vi "WebDAV write.vi"(0 "RIO Filepath":path, 5 "CA Number":string, 7 "Test Name":string, 9 "Date":string, 11 "Filename":string) -> (15 "error out":errorcluster)   [LabVIEW 2019]
uses:
  <vilib>/WebDAVClient/Advanced/Put File.vi
  <vilib>/WebDAVClient/NI_WebDAV.lvlib
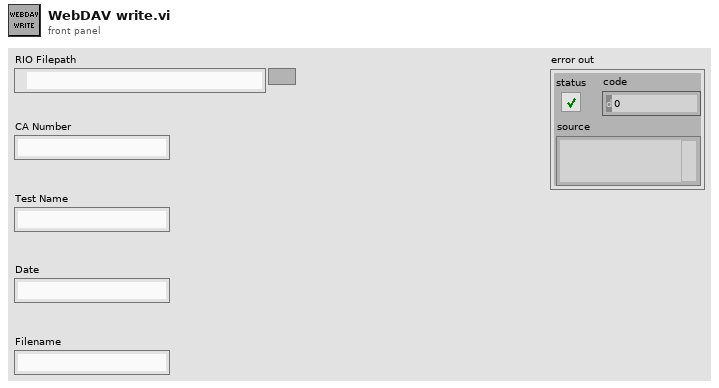
[diagram p1: front panel]
types:
  T1 = typedef "NI_WebDAV.lvlib/SessionHandle.ctl" = refnum<k1>
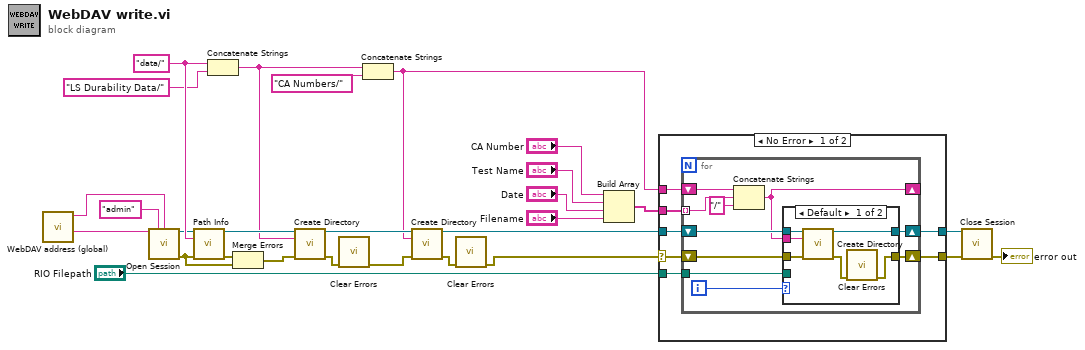
[diagram p0: block diagram]
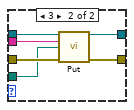
[diagram p2: hidden frame]
diagram:
  w28 = "data/" ("relative uri")
  n1 = call "WebDAV address (global).vi"() -> ("Password OUT"=w13:string, "WebDAV Address"=w12:string)  [unwired: 8 in]
  n2 = call <vilib>:"Open Session.vi"("host uri prefix"=w12, "username"="admin", "password"=w13) -> ("session handle out"=w24:T1, "error out"=w22:errorcluster)  [unwired: 11 in]
  n3 = call <vilib>:"Path Info.vi"("session handle"=w24, "relative uri"=w28, "error in (no error)"=w22) -> ("session handle out"=w7:T1, "error out"=w23:errorcluster)  [unwired: 9 in, 2 out]
  n4 = Concatenate Strings(w28, "LS Durability Data/" ("relative uri")) -> (w2:string)
  n5 = Merge Errors(w23, w22) -> (w6:errorcluster)
  n6 = call <vilib>:"Create Directory.vi"("session handle"=w7, "relative uri"=w2, "error in (no error)"=w6) -> ("session handle out"=w8:T1, "error out"=w11:errorcluster)  [unwired: 11 in]
  n7 = call <vilib>:"Clear Errors.vi"("error in (no error)"=w11) -> ("error out"=w9:errorcluster)  [unwired: 5 in, 1 out]
  n8 = Concatenate Strings(w2, "CA Numbers/" ("relative uri")) -> (w1:string)
  n9 = call <vilib>:"Create Directory.vi"("session handle"=w8, "relative uri"=w1, "error in (no error)"=w9) -> ("session handle out"=w4:T1, "error out"=w10:errorcluster)  [unwired: 11 in]
  n10 = call <vilib>:"Clear Errors.vi"("error in (no error)"=w10) -> ("error out"=w5:errorcluster)  [unwired: 5 in, 1 out]
  n11 = Build Array("CA Number", "Test Name", "Date", "Filename") -> (w18:string[])
  n12 = case shown="No Error" w5 {
    selector: w5 -> [w35 w59]
    tunnel: w4 -> [w34 w58]
    tunnel: [w31 w58] -> w25
    tunnel: [w30 w59] -> w26
    tunnel: w1 -> [w33 _]
    tunnel: w18 -> [w32 _]
    tunnel: "RIO Filepath" -> [w29 _]
    frame No Error {
      n13 = for {
        shift-right: [w40] -> _
        shift-left: w33 -> [w45]
        shift-right: [w41] -> w31
        shift-left: w34 -> [w42]
        shift-right: [w39] -> w30
        shift-left: w35 -> [w38]
        tunnel: w32 -> [w44] mode=indexing
        tunnel: w29 -> [w36]
        i -> [w37]
        n14 = Concatenate Strings(w45, w44, "/" ("string")) -> (w40:string)
        n15 = case shown="Default" w37 {
          tunnel: w42 -> [w51 w57]
          tunnel: [w50 w56] -> w41
          tunnel: w40 -> [w49 w55]
          tunnel: [w47 w53] -> w39
          tunnel: w38 -> [w46 w54]
          tunnel: w36 -> [_ w52]
          frame Default {
            n16 = call <vilib>:"Create Directory.vi"("session handle"=w51, "relative uri"=w49, "error in (no error)"=w46) -> ("session handle out"=w50:T1, "error out"=w48:errorcluster)  [unwired: 11 in]
            n17 = call <vilib>:"Clear Errors.vi"("error in (no error)"=w48) -> ("error out"=w47:errorcluster)  [unwired: 5 in, 1 out]
          }
          frame 3 {
            n18 = call-poly <vilib>:"Put.vi"("session handle"=w57, "relative uri"=w55, "local file path"=w52, "error in (no error)"=w54) -> ("session handle out"=w56:T1, "error out"=w53:errorcluster)  [unwired: 9 in, 1 out]
          }
        }
      }
    }
    frame Error {
    }
  }
  n19 = call <vilib>:"Close Session.vi"("session handle"=w25, "error in (no error)"=w26) -> ("error out"=→"error out":errorcluster)  [unwired: 13 in]
